vi "Chronos TDMS Find Files in Time Range.vi"(8 "error in (no error)":errorcluster, 9 "Scale":T2, 10 "Time Ranges":T1, 11 "TDMS Files":path[](array[path])) -> (0 "error out":errorcluster, 3 "Files out":path[](array[path]))   [LabVIEW 2021]
uses:
  <vilib>/Utility/miscctls.llb/LVRangeTypeDef.ctl
  typedefs/Chronos cluster Time Ranges.ctl
panel:
  out "time stamp 2":timestamp
  out "time stamp":timestamp
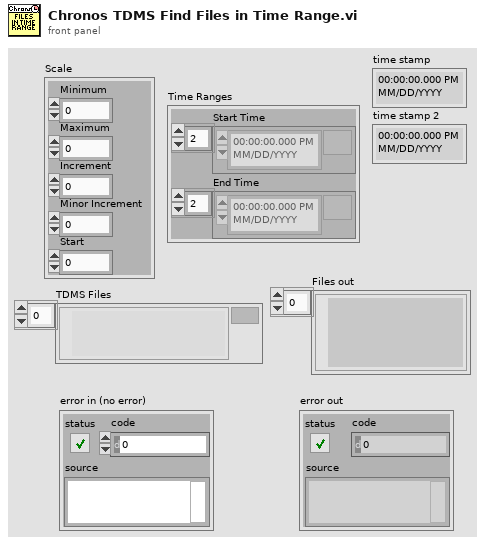
[diagram p1: front panel]
types:
  T1 = typedef "Chronos cluster Time Ranges.ctl" = cluster{"Start Time":timestamp[], "End Time":timestamp[]}
  T2 = typedef "LVRangeTypeDef.ctl" = cluster{"Minimum":dbl, "Maximum":dbl, "Increment":dbl, "Minor Increment":dbl, "Start":dbl}
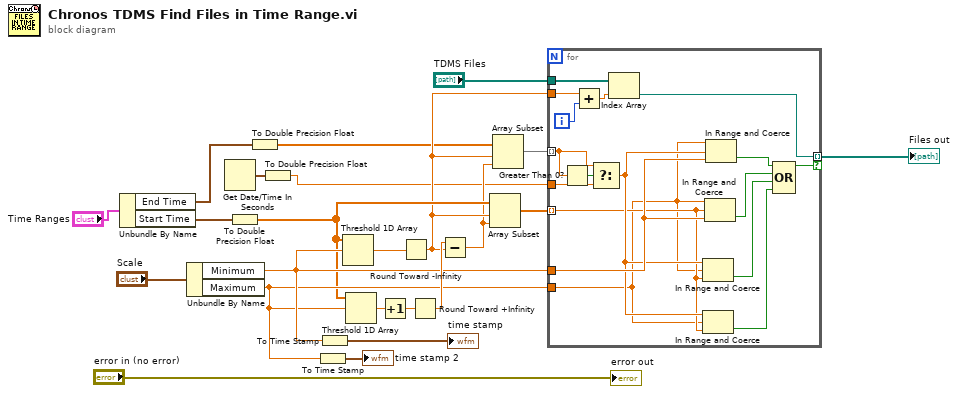
[diagram p0: block diagram]
diagram:
  n1 = Unbundle By Name("Time Ranges") -> ("End Time"=w7:timestamp[], "Start Time"=w8:timestamp[])
  n2 = Unbundle By Name("Scale") -> ("Minimum"=w12:dbl, "Maximum"=w11:dbl)
  n3 = Get Date/Time In Seconds() -> (seconds since 1Jan1904=w2:timestamp)
  n4 = To Double Precision Float(number=w8) -> (double precision float=w10:dbl[])
  n5 = To Double Precision Float(number=w7) -> (double precision float=w3:dbl[])
  n6 = To Double Precision Float(number=w2) -> (double precision float=w1:dbl)
  n7 = To Time Stamp(1:w11) -> (0:→"time stamp 2":timestamp)
  n8 = To Time Stamp(1:w12) -> (0:→"time stamp":timestamp)
  n9 = Threshold 1D Array(2:w12, 3:w10) -> (0:w19:dbl)  [unwired: 1 in]
  n10 = Threshold 1D Array(2:w11, 3:w10) -> (0:w20:dbl)  [unwired: 1 in]
  n11 = Increment(x=w20) -> (x+1=w15:dbl)
  n12 = Round Toward -Infinity(1:w19) -> (0:w6:dbl)
  n13 = Round Toward +Infinity(x=w15) -> (ceil(x): smallest int >= x=w18:dbl)
  n14 = Subtract(x=w18, y=w6) -> (x-y=w5:dbl)
  n15 = Array Subset(array=w10, index=w6, length=w5) -> (w14:dbl[])
  n16 = Array Subset(array=w3, index=w6, length=w5) -> (w4:dbl[])
  n17 = for {
    tunnel: w14 -> [w27] mode=indexing
    tunnel: "TDMS Files" -> [w40]
    tunnel: w6 -> [w39]
    tunnel: [w36] -> w9 mode=indexing if=w34
    tunnel: w12 -> [w29]
    tunnel: w11 -> [w26]
    tunnel: w4 -> [w31] mode=indexing
    tunnel: w1 -> [w30]
    i -> [w38]
    n18 = Greater Than 0?(x=w31) -> (x > 0?=w32:bool)
    n19 = Add(x=w39, y=w38) -> (x+y=w37:dbl)
    n20 = Select(t=w31, s=w32, f=w30) -> (s? t:f=w28:dbl)
    n21 = Index Array(array=w40, index=w37) -> (element=w36:path)
    n22 = In Range and Coerce(upper limit=w28, x=w26, lower limit=w27) -> (In Range?=w25:bool)  [unwired: 1 out]
    n23 = In Range and Coerce(upper limit=w28, x=w26, lower limit=w27) -> (In Range?=w24:bool)  [unwired: 1 out]
    n24 = In Range and Coerce(upper limit=w26, x=w27, lower limit=w29) -> (In Range?=w35:bool)  [unwired: 1 out]
    n25 = In Range and Coerce(upper limit=w26, x=w28, lower limit=w29) -> (In Range?=w33:bool)  [unwired: 1 out]
    n26 = Compound Arithmetic op=OR(w33, w35, w25, w24) -> (w34:bool)
  }
  "Files out" <- w9
  "error out" <- "error in (no error)"
